vi "X_2.87_Varme_med_passiv_koling.vi"() -> ()   [LabVIEW 2022 SP3]
uses:
  <extravilib>/ChannelInstances/Tag-c(dbl,dbl,dbl)/Write With Abort.vi
  <extravilib>/ChannelInstances/Tag-bool/Write With Abort.vi
  <extravilib>/ChannelInstances/Stream-dbl/Read With Abort.vi
  <extravilib>/ChannelInstances/Tag-bool/Read With Abort.vi
  <extravilib>/ChannelInstances/Tag-c(dbl,dbl,dbl)/Read With Abort.vi
  <extravilib>/ChannelInstances/Stream-dbl/Write With Abort.vi
  <extravilib>/ChannelInstances/Stream-dbl/EndpointRead.vi
  <extravilib>/ChannelInstances/Stream-dbl/Endpoint.vi
  <extravilib>/ChannelInstances/Tag-c(dbl,dbl,dbl)/Instantiate.vi
  <extravilib>/ChannelInstances/Tag-c(dbl,dbl,dbl)/Endpoint.vi
  <extravilib>/ChannelInstances/Stream-dbl/Instantiate.vi
  <extravilib>/ChannelInstances/Tag-bool/Instantiate.vi
  <extravilib>/ChannelInstances/Stream-dbl/)Channel.vi
  <resource>/ChannelSupport/_ChannelSupport/WaitIfNeeded.vi
  <extravilib>/ChannelInstances/Tag-bool/EndpointRead.vi
  <extravilib>/ChannelInstances/Tag-c(dbl,dbl,dbl)/EndpointRead.vi
  <extravilib>/ChannelInstances/Tag-bool/Endpoint.vi
  <extravilib>/ChannelInstances/Stream-dbl.lvlib
  <extravilib>/ChannelInstances/Tag-c(dbl,dbl,dbl).lvlib
  <extravilib>/ChannelInstances/Tag-bool.lvlib
panel:
  out "Boolean 2":bool
  in  "Boolean":bool
  in  "Coerce?":bool
  out "u":dbl
  in  "Regulation type":T1(ring)
  in  "k_d":dbl
  in  "k_i":dbl
  in  "k_p":dbl
  in  "SP":dbl
  out "Iteration tid (s)":dbl
  out "Heater %":dbl
  out "Fan %":dbl
  out "Numeric 3":i32
  in  "Default values":T2={"heater effect"=10.0, "Cp"=10.0, "masse"=10.0, "Iteration tid (s)"=0.0, "Default temp"=20.0}
  out "temp chart":dbl(graph)
  in  "UI Cluster":T3={"Amb Temp"=24.484536082474225, "Fan %"=100.0, "Heater %"=99.88297024147607} {"Heater %" scale=0.0..100.0; "Fan %" scale=0.0..100.0; "Amb Temp" scale=0.0..50.0}
  out "Numeric 2":i32
  out "Numeric":i32
  out "Temp":dbl
  in  "stop":bool
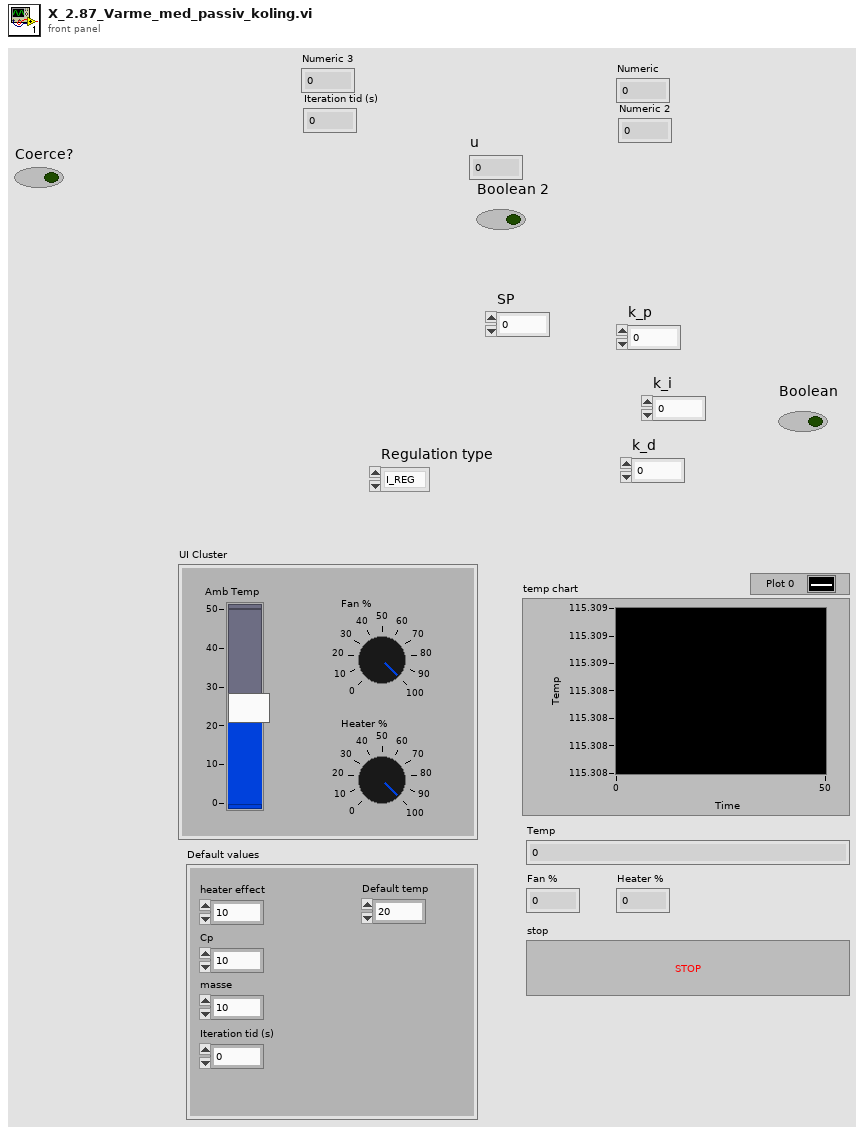
[diagram p1: front panel]
types:
  T1 = enum16{"I_REG", "ID_REG", "P_REG", "PI_REG", "PD_REG", "PID_REG"}
  T2 = cluster{"heater effect":dbl, "Cp":dbl, "masse":dbl, "Iteration tid (s)":dbl, "Default temp":dbl}
  T3 = cluster{"Amb Temp":dbl, "Fan %":dbl, "Heater %":dbl}
  T4 = typedef "Tag-c(dbl,dbl,dbl).lvlib/))Channel.ctl" = refnum<queue>
  T5 = typedef "Tag-bool.lvlib/))Channel.ctl" = refnum<queue>
  T6 = typedef "Stream-dbl.lvlib/)Channel.ctl" = refnum<queue>
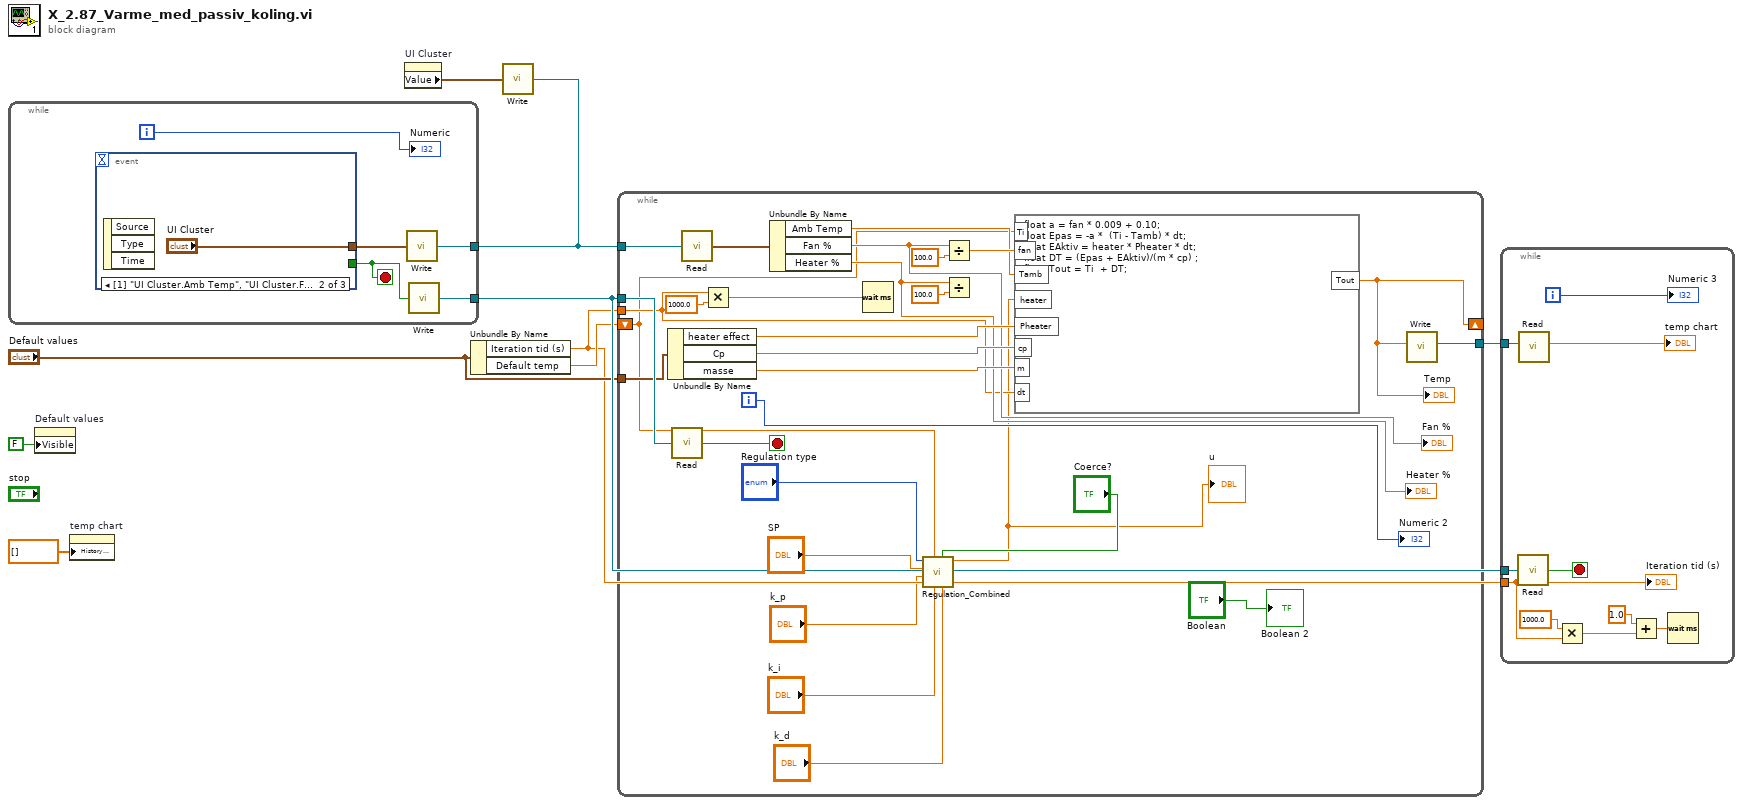
[diagram p0: block diagram]
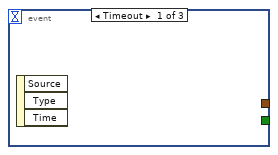
[diagram p2: hidden frame]
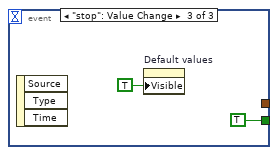
[diagram p3: hidden frame]
diagram:
  n1 = while {
    tunnel: [w14] -> w9
    tunnel: [w10] -> w7
    i -> [w13]
    stop <- w12 stop-if-true
    n2 = event shown="[1] \"UI Cluster.Amb Temp\", \"UI Cluster.Fan %\", \"UI Cluster.Heater %\": Value Change" {
      selector: _ -> [_ _ _]
      dyn-events: _ -> [_ _ _]
      timeout: _ -> [_ _ _]
      tunnel: [_ _ TRUE ("stop")] -> w12
      tunnel: [_ "UI Cluster" _] -> w11
      event Timeout {
        n3 = event-data() -> ()  [unwired: 1 in, 3 out]
      }
      event "UI Cluster.Amb Temp", "UI Cluster.Fan %", "UI Cluster.Heater %": Value Change {
        n4 = event-data() -> ()  [unwired: 1 in, 3 out]
      }
      event "stop": Value Change {
        n5 = event-data() -> ()  [unwired: 1 in, 3 out]
        n6 = property on="Default values" class="Clust (strict)"("Visible"=TRUE) -> ()  [unwired: 2 in, 2 out]
      }
    }
    n7 = call <extravilib>:"Write.vi"("element"=w11) -> ("channel"=w10:T4)  [unwired: 1 out]
    n8 = call <extravilib>:"Write.vi"("element"=w12) -> ("channel"=w14:T5)  [unwired: 1 out]
    "Numeric" <- w13
  }
  n9 = property on="Default values" class="Clust (strict)"("Visible"=FALSE) -> ()  [unwired: 2 in, 2 out]
  n10 = property on="temp chart" class="WFChart (strict)"("History Data"=dbl[] []) -> ()  [unwired: 2 in, 2 out]
  n11 = property on="UI Cluster" class="Clust (strict)"() -> ("Value"=w6:T3)  [unwired: 2 in, 2 out]
  n12 = Unbundle By Name("Default values") -> ("Iteration tid (s)"=w1:dbl, "Default temp"=w2:dbl)
  n13 = call <extravilib>:"Write.vi"("element"=w6, "channel"=w7) -> ()  [unwired: 1 out]
  n14 = while {
    shift-right: [w46] -> _
    shift-left: w2 -> [w25]
    tunnel: w9 -> [w45]
    tunnel: [w42] -> w8
    tunnel: w7 -> [w32]
    tunnel: "Default values" -> [w28]
    tunnel: w1 -> [w27]
    i -> [w43]
    stop <- w44 stop-if-true
    n15 = Unbundle By Name(w28) -> ("heater effect"=w41:dbl, "Cp"=w40:dbl, "masse"=w39:dbl)
    n16 = call <extravilib>:"Read.vi"("channel"=w45) -> ("element"=w44:bool)  [unwired: 1 in, 1 out]
    n17 = call <extravilib>:"Read.vi"("channel"=w32) -> ("element"=w31:T3)  [unwired: 1 in, 1 out]
    n18 = Multiply(x=w27, y=1000.0) -> (x*y=w37:dbl)
    n19 = Unbundle By Name(w31) -> ("Amb Temp"=w33:dbl, "Fan %"=w30:dbl, "Heater %"=w29:dbl)
    "Fan %" <- w30
    "Heater %" <- w29
    n20 = Wait (ms)(milliseconds to wait=w37) -> ()  [unwired: 1 out]
    n21 = call "Regulation_Combined.vi"("k_d"="k_d", "Coerce?"="Coerce?", "k_i"="k_i", "DATA"=w25, "k_p"="k_p", "SP"="SP", "Regulation type"="Regulation type") -> ("u"=w19:dbl)  [unwired: 4 in]
    "u" <- w19
    n22 = Divide(x=w30, y=100.0) -> (x/y=w34:dbl)
    n23 = Divide(x=w29, y=100.0) -> ()  [unwired: 1 out]
    n24 = formula code="float a = fan * 0.009 + 0.10;\nfloat Epas = -a *  (Ti - Tamb) * dt;\nfloat EAktiv = heater * Pheater * dt;\nfloat DT = (Epas + EAktiv)/(m * cp) ;\nfloat Tout = Ti  + DT;"("Tamb"=w33, "fan"=w34, "Ti"=w25, "dt"=w27, "cp"=w40, "m"=w39, "heater"=w19, "Pheater"=w41) -> ("Tout"=w46:dbl)
    "Temp" <- w46
    n25 = call <extravilib>:"Write.vi"("element"=w46) -> ("channel"=w42:T6)  [unwired: 8 in, 2 out]
    "Numeric 2" <- w43
    "Boolean 2" <- "Boolean"
  }
  n26 = while {
    tunnel: w9 -> [w56]
    tunnel: w8 -> [w55]
    tunnel: w1 -> [w50]
    i -> [w53]
    stop <- w52 stop-if-true
    n27 = call <extravilib>:"Read.vi"("channel"=w56) -> ("element"=w52:bool)  [unwired: 1 in, 1 out]
    n28 = call <extravilib>:"Read.vi"("channel"=w55) -> ("element"=→"temp chart":dbl)  [unwired: 6 in, 4 out]
    n29 = Multiply(x=1000.0 ("y"), y=w50) -> (x*y=w48:dbl)
    n30 = Add(x=1.0, y=w48) -> (x+y=w47:dbl)
    n31 = Wait (ms)(milliseconds to wait=w47) -> ()  [unwired: 1 out]
    "Numeric 3" <- w53
    "Iteration tid (s)" <- w50
  }
